vi "Write then read.vi"(7 "Max bytes to read (999)":u32=999, 8 "error in (no error)":errorcluster, 9 "Trim RX? (T)":bool, 10 "TX Data":string, 11 "Serial Device in":refnum<class "Serial Device.lvclass">) -> (0 "error out":errorcluster, 2 "RX Data":string, 3 "Serial Device out":refnum<class "Serial Device.lvclass">)   [LabVIEW 2019, in "Serial Device.lvclass"]
uses:
  Serial Device.lvclass
  Serial Device.lvclass/Serial Device.ctl
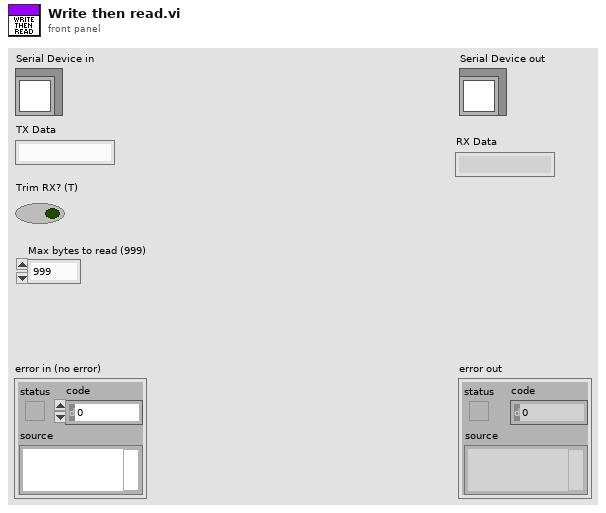
[diagram p1: front panel]
types:
  T1 = typedef "Semaphore RefNum" = refnum<k1>
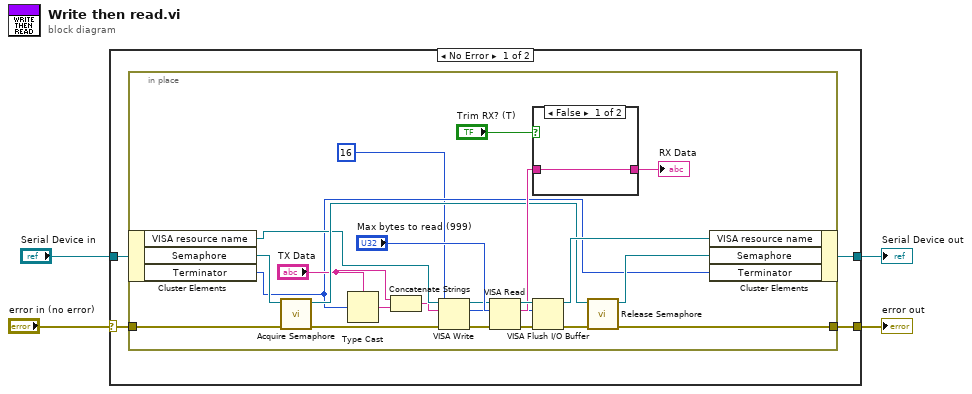
[diagram p0: block diagram]
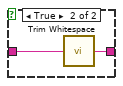
[diagram p2: hidden frame]
diagram:
  n1 = case shown="No Error" "error in (no error)" {
    selector: "error in (no error)" -> [w8 w35]
    tunnel: [w5 w35] -> w3
    tunnel: [w6 w34] -> w1
    tunnel: "Serial Device in" -> [w7 w34]
    frame No Error {
      n2 = in-place {
        in-place-border: w8 -> [w29]
        in-place-border: [w19] -> w5
        n3 = in-place-cluster #1(w7) -> ("VISA resource name"=w14:refnum<visa-resource-name>, "Semaphore"=w28:T1, "Terminator"=w10:u8)
        n4 = call <vilib>:"Acquire Semaphore.vi"("error in (no error)"=w29, "semaphore"=w28) -> ("error out"=w17:errorcluster, "semaphore out"=w20:T1)  [unwired: 3 in, 1 out]
        n5 = Type Cast(type="TX Data", x=w10) -> (*(type *) &x=w11:string)
        n6 = Concatenate Strings("TX Data", w11) -> (w13:string)
        n7 = VISA Write(VISA resource name=w14, write buffer=w13, error in (no error)=w17) -> (VISA resource name out=w15:refnum<visa-resource-name>, error out=w16:errorcluster)  [unwired: 1 out]
        n8 = VISA Read(VISA resource name=w15, byte count="Max bytes to read (999)", error in (no error)=w16) -> (VISA resource name out=w27:refnum<visa-resource-name>, read buffer=w24:string, error out=w22:errorcluster)  [unwired: 1 out]
        n9 = case shown="False" "Trim RX? (T)" {
          tunnel: [w31 w33] -> w25
          tunnel: w24 -> [w31 w32]
          frame False {
          }
          frame True {
            n10 = call <vilib>:"Trim Whitespace.vi"("string"=w32) -> ("trimmed string"=w33:string)  [unwired: 1 in]
          }
        }
        "RX Data" <- w25
        n11 = VISA Flush I/O Buffer(VISA resource name=w27, mask (16)=16, error in (no error)=w22) -> (VISA resource name out=w26:refnum<visa-resource-name>, error out=w23:errorcluster)
        n12 = call <vilib>:"Release Semaphore.vi"("error in (no error)"=w23, "semaphore"=w20) -> ("error out"=w19:errorcluster, "semaphore out"=w21:T1)  [unwired: 4 in]
        n13 = in-place-cluster #1("VISA resource name"=w26, "Semaphore"=w21, "Terminator"=w10) -> (w6:refnum<class "Serial Device.lvclass">)
      }
    }
    frame Error {
    }
  }
  "error out" <- w3
  "Serial Device out" <- w1
